vi "load_single_image.vi"(8 "error in (no error)":errorcluster, 11 "data_loader_single_image in":refnum<class "data_loader_single_image.lvclass">) -> (0 "error out":errorcluster, 3 "data_loader_single_image out":refnum<class "data_loader_single_image.lvclass">)   [LabVIEW 2017, in "data_loader_single_image.lvclass"]
uses:
  data_loader_single_image.lvclass
  data_loader_single_image.lvclass/data_loader_single_image.ctl
panel:
  out "record the secondary name":bool
  out "secondary list":string[](array[string])
  in  "error in":errorcluster
  out "error out 2":errorcluster
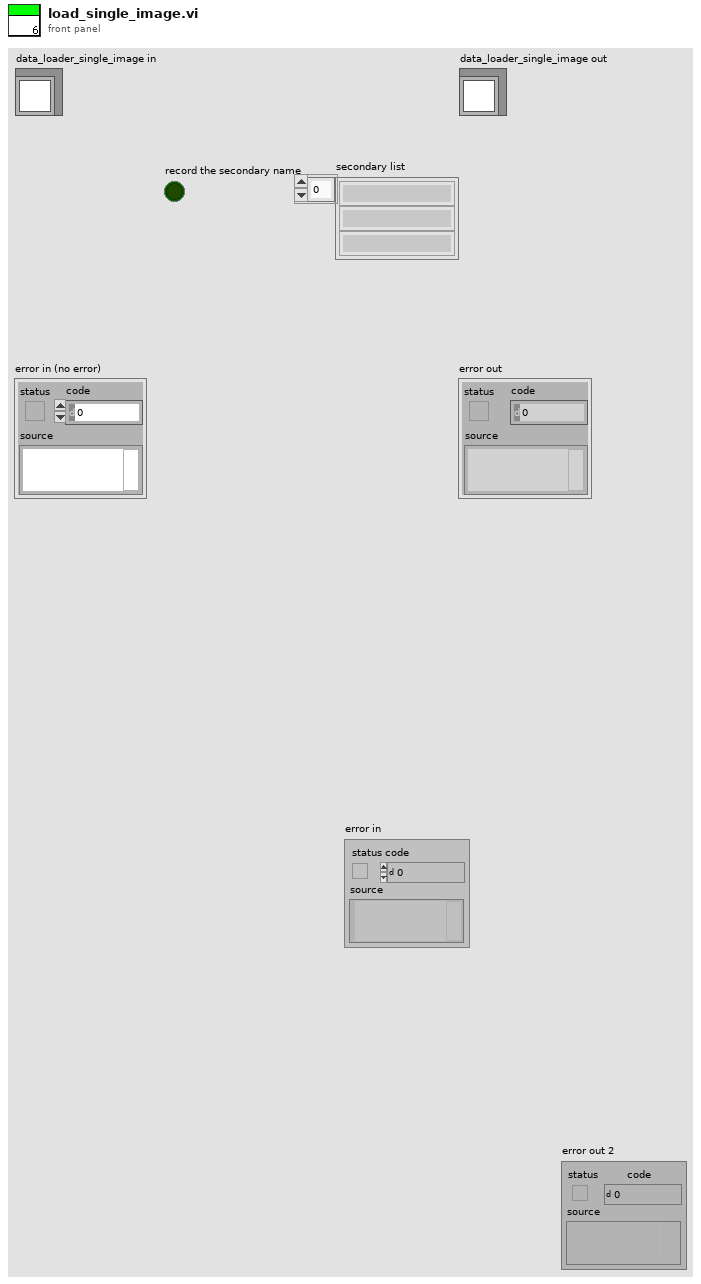
[diagram p1: front panel]
types:
  T1 = typedef "IMAQ Image.ctl" = refnum<image>
  T2 = typedef "Image Type" = u32
  T3 = typedef "imagedata.ctl" = cluster{"image type":i32, "image depth":i32, "image":u8[], "mask":u8[], "colors":u32[], "Rectangle":cluster{"left":i16, "top":i16, "right":i16, "bottom":i16}}
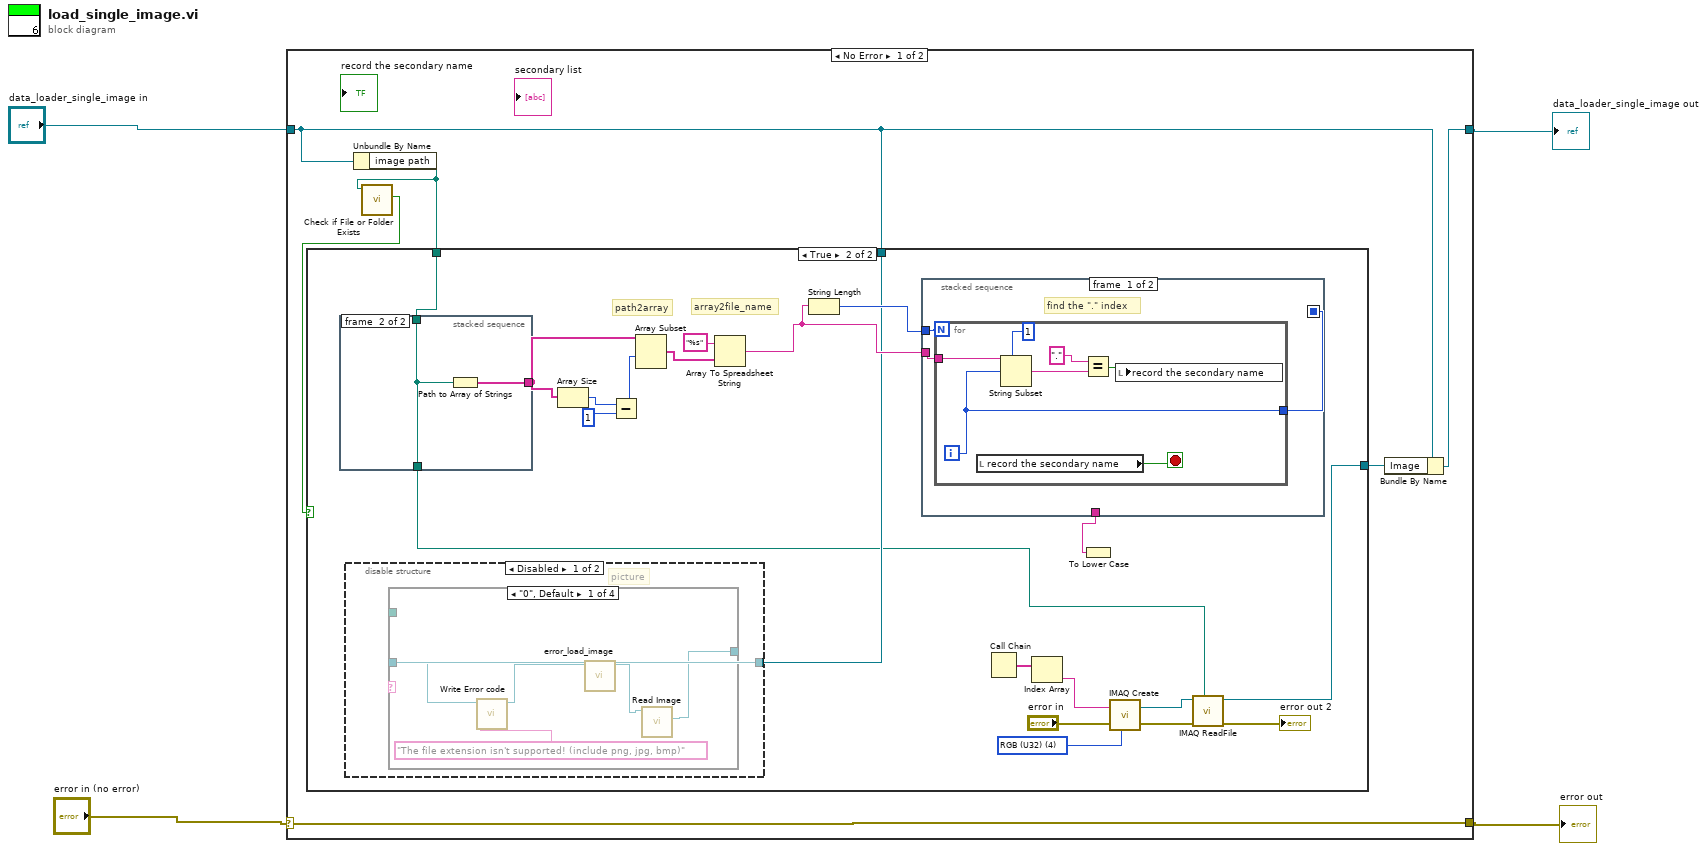
[diagram p0: block diagram]
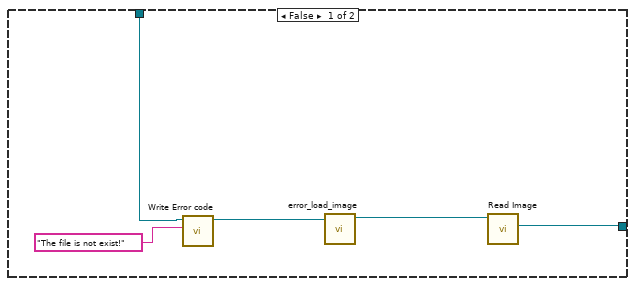
[diagram p2: hidden frame]
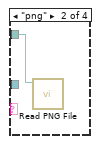
[diagram p3: hidden frame]
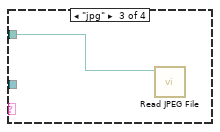
[diagram p4: hidden frame]
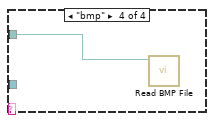
[diagram p5: hidden frame]
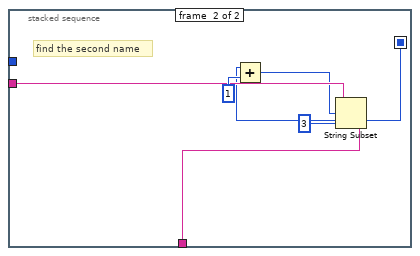
[diagram p7: hidden frame]
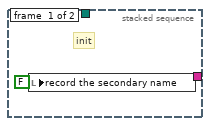
[diagram p8: hidden frame]
diagram:
  n1 = case shown="No Error" "error in (no error)" {
    selector: "error in (no error)" -> [w10 w66]
    tunnel: [w10 w66] -> w2
    tunnel: [w9 w65] -> w1
    tunnel: "data_loader_single_image in" -> [w8 w65]
    frame No Error {
      n2 = Unbundle By Name(w8) -> ("image path"=w7:path)
      n3 = call <vilib>:"Check if File or Folder Exists.vi"("path"=w7) -> ("file or folder exists?"=w6:bool)  [unwired: 8 in, 2 out]
      n4 = case shown="True" w6 {
        tunnel: w8 -> [w14 w26]
        tunnel: w7 -> [_ w25]
        tunnel: [w11 w17] -> w5
        frame False {
          n5 = call-dynamic "Write Error code.vi"("Error code"="The file is not exist!", "data_loader in"=w14) -> ("data_loader out"=w13:refnum<class "data_loader_single_image.lvclass">)  [unwired: 8 in, 1 out]
          n6 = call-dynamic "error_load_image.vi"("data_loader in"=w13) -> ("data_loader out"=w12:refnum<class "data_loader_single_image.lvclass">)  [unwired: 9 in, 1 out]
          n7 = call-dynamic "Read Image .vi"("data_loader in"=w12) -> ("Image"=w11:T1)  [unwired: 8 in, 2 out]
        }
        frame True {
          w20 = T2 4 items=["Grayscale (U8)", "Grayscale (I16)", "Grayscale (SGL)", "Complex (CSG)", "RGB (U32)", "HSL (U32)", "RGB (U64)", "Grayscale (U16)"] ("Image Type")
          # "array2file_name"
          # "path2array"
          n8 = stacked-sequence {
            tunnel: w25 -> [_ w63]
            tunnel: [_ w64] -> w27
            tunnel: [_ w63] -> w16
            frame #0 {
              # "init"
              n9 = local write "record the secondary name"(FALSE) -> ()
            }
            frame #1 {
              n10 = Path to Array of Strings(0:w63) -> (2:w64:string[])  [unwired: 1 out]
            }
          }
          n11 = disable-structure shown="Disabled" {
            disable-tunnel: w26 -> [w36 _]
            frame Disabled {
              # "picture"
              n12 = case shown="\"0\", Default" {
                selector: _ -> [_ _ _ _]
                tunnel: _ -> [_ w42 w43 w44]
                tunnel: [w37 _ _ _] -> _
                tunnel: w36 -> [w40 _ _ _]
                frame "0", Default {
                  n13 = call-dynamic "Write Error code.vi"("Error code"="The file extension isn't supported! (include png, jpg, bmp)", "data_loader in"=w40) -> ("data_loader out"=w39:refnum<class "data_loader_single_image.lvclass">)  [unwired: 8 in, 1 out]
                  n14 = call-dynamic "error_load_image.vi"("data_loader in"=w39) -> ("data_loader out"=w38:refnum<class "data_loader_single_image.lvclass">)  [unwired: 9 in, 1 out]
                  n15 = call-dynamic "Read Image .vi"("data_loader in"=w38) -> ("Image"=w37:T1)  [unwired: 8 in, 2 out]
                }
                frame "png" {
                  n16 = call <vilib>:"Read PNG File.vi"("path to PNG file"=w42) -> ()  [unwired: 8 in, 3 out]
                }
                frame "jpg" {
                  n17 = call <vilib>:"Read JPEG File.vi"("path to JPEG file"=w43) -> ()  [unwired: 8 in, 3 out]
                }
                frame "bmp" {
                  n18 = call <vilib>:"Read BMP File.vi"("path to BMP file"=w44) -> ("image data"=w45:T3)  [unwired: 8 in, 2 out]
                }
              }
            }
            frame Enabled {
            }
          }
          n19 = Array Size(array=w27) -> (size(s)=w34:i32)
          n20 = Subtract(x=w34, y=1) -> (x-y=w33:i32)
          n21 = Array Subset(array=w27, index=w33) -> (w32:string[])  [unwired: 1 in]
          n22 = Array To Spreadsheet String(array=w32, 3:"%s" ("format string")) -> (spreadsheet string=w30:string)  [unwired: 1 in]
          n23 = String Length(string=w30) -> (length=w29:i32)
          n24 = stacked-sequence {
            seq-local: [w46 _] -> [_ w57]
            tunnel: w30 -> [w48 w59]
            tunnel: w29 -> [w47 _]
            tunnel: [_ w60] -> w28
            frame #0 {
              # "find the \".\" index"
              n25 = for {
                N: w47 -> [_]
                tunnel: w48 -> [w55]
                tunnel: [w49] -> w46
                i -> [w49]
                stop <- w50 stop-if-true
                n26 = local read "record the secondary name"() -> (w50:bool)
                n27 = String Subset(string=w55, offset (0)=w49, length (rest)=1 ("length (rest)")) -> (substring=w51:string)
                n28 = Equal?(x=".", y=w51) -> (x = y?=w52:bool)
                n29 = local write "record the secondary name"(w52) -> ()
              }
            }
            frame #1 {
              # "find the second name"
              n30 = Add(x=w57, y=1) -> (x+y=w58:i32)
              n31 = String Subset(string=w59, offset (0)=w58, length (rest)=3) -> (substring=w60:string)
            }
          }
          n32 = Call Chain() -> (call chain=w22:string[])
          n33 = Index Array(array=w22) -> (element=w21:string)  [unwired: 1 in]
          n34 = To Lower Case(string=w28) -> ()  [unwired: 1 out]
          n35 = call "IMAQ Create"("Image Name"=w21, "Image Type"=w20, "error in (no error)"="error in") -> ("New Image"=w19:T1, "error out"=w24:errorcluster)  [unwired: 1 in, 1 out]
          n36 = call "IMAQ ReadFile"("File Path"=w16, "error in (no error)"=w24, "Image"=w19) -> ("error out"=→"error out 2":errorcluster, "Image Out"=w17:T1)  [unwired: 2 in, 5 out]
        }
      }
      n37 = Bundle By Name(cluster=w8, "Image"=w5) -> (w9:refnum<class "data_loader_single_image.lvclass">)
    }
    frame Error {
    }
  }
  "error out" <- w2
  "data_loader_single_image out" <- w1
